vi "Analysis.vi"() -> ()   [LabVIEW 2020]
doc: "Use this template to simulate the generation and display of data.\nNote: LabVIEW enables automatic error handling by default for VIs you create from this template."
uses:
  Instance           1 27Saved   GenerateDisplay.vit .vi
  <vilib>/express/express shared/transition.llb/Dynamic To Waveform Array.vi
  <vilib>/express/express arith-compare/Formula/Block/exnFormulaBlock how many pts in the wave.vi
  <vilib>/express/express shared/ex_Modify Signal Name.vi
  <vilib>/express/express shared/transition.llb/Waveform Array To Dynamic.vi
  <vilib>/measure/mascope.llb/Amplitude and Levels N chan.vi
  <vilib>/express/express arith-compare/Formula/XNode/ExpressFormulaBlockNode.xnode
  <vilib>/measure/NI_MAPro.lvlib
panel:
  in  "Amplitude":dbl(knob) scale=0.0..10.0
  out "Warning":bool
  out "Peak value":dbl
  out "low state level":dbl[](array[numeric]) format="%.2p"
  out "high state level":dbl[](array[numeric]) format="%.2p"
  out "amplitude":dbl[](array[numeric]) format="%.2p"
  out "Filtered Graph":dynamicdata(graph)
  out "Unfiltered Graph":dynamicdata(graph)
  in  "stop":bool
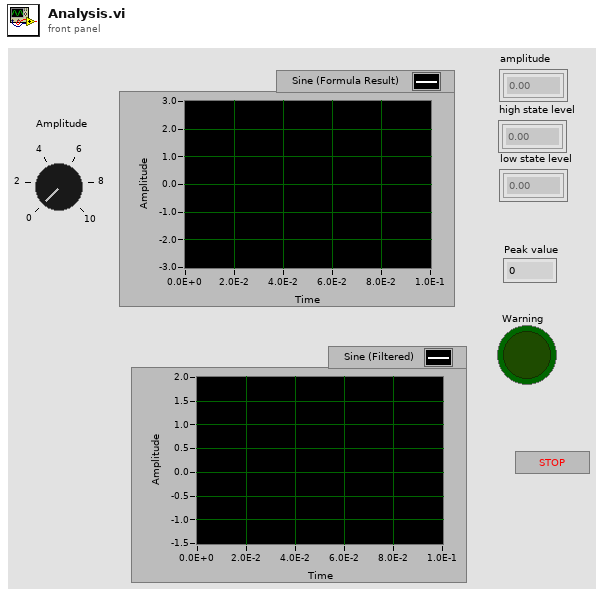
[diagram p1: front panel]
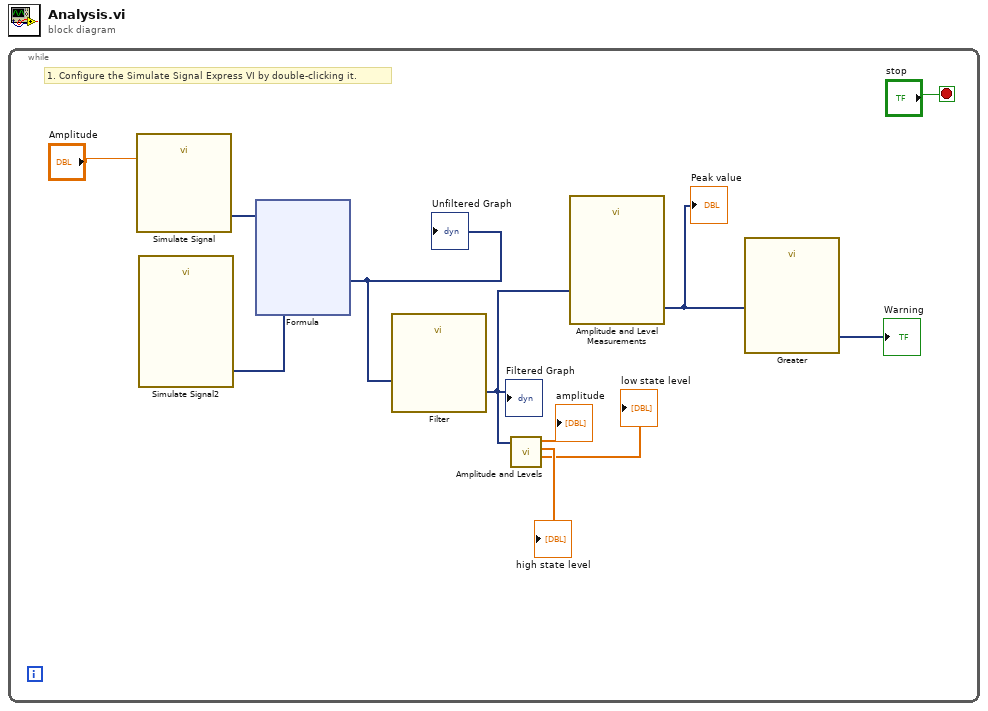
[diagram p0: block diagram]
diagram:
  n1 = while {
    stop <- "stop" stop-if-true
    # "1. Configure the Simulate Signal Express VI by double-clicking it."
    n2 = call "Simulate Signal"("Amplitude"="Amplitude") -> ("Sine"=w10:dynamicdata)  [unwired: 13 in, 1 out]
    n3 = call "Simulate Signal2"() -> ("60Hz and noise"=w9:dynamicdata)  [unwired: 14 in, 1 out]
    n4 = xnode "Formula"("Sine"=w10, "Noise"=w9) -> ("Result"=w8:dynamicdata)  [unwired: 1 in, 1 out]
    "Unfiltered Graph" <- w8
    n5 = call "Filter"("Signal"=w8) -> ("Filtered Signal"=w4:dynamicdata)  [unwired: 9 in, 1 out]
    "Filtered Graph" <- w4
    n6 = call-poly <vilib>:"Amplitude and Levels.vi"("signal(s) in"=w4) -> ("low state level"=→"low state level":dbl[], "high state level"=→"high state level":dbl[], "amplitude"=→"amplitude":dbl[])  [unwired: 7 in, 1 out]
    n7 = call "Amplitude and Level Measurements"("Signals"=w4) -> ("Peak to Peak"=w1:dynamicdata)  [unwired: 13 in, 1 out]
    "Peak value" <- w1
    n8 = call "Greater"("Operand 1"=w1) -> ("Result"=→"Warning":dynamicdata)  [unwired: 9 in, 1 out]
  }
